vi "Dot_Plot_Sub.vi"(8 "Scaler plotted":string, 11 "Data":dbl[][](array[numeric])=[[-106.4208, 283.2907, 10.0, -0.027074, 202.4772, -73.9844, 9.9544], [-106.4108, 183.2989, 10.0, -0.06373, 202.4772, -73.9844, 9.9544], [-106.4104, 233.2978, 10.0, -0.10129, 202.4772, -73.9844, 9.9544], [-106.408, 333.302, 10.0, -0.09306, 202.4772, -73.9844, 9.9544], [138.8906, 606.731, 10.0, -0.003285, 202.4772, -73.9844, 9.9544], [238.889, 47.6577, 10.0, 0.004673, 202.4772, -73.9844, 9.9544], [238.8902, 606.729, 10.0, -0.003458, 202.4772, -73.9844, 9.9544], [288.8878, 47.6581, 10.0, 0.007221, 202.4772, -73.9844, 9.9544], [338.888, 606.73, 10.0, 0.004362, 202.4772, -73.9844, 9.9544], [338.891, 47.6626, 10.0, 0.006298, 202.4772, -73.9844, 9.9544], [388.892, -63.3583, 10.0, 4.5324, 202.4772, -73.9844, 9.9544], [388.892, 47.6606, 10.0, -0.008191, 202.4772, -73.9844, 9.9544], [438.889, 606.729, 10.0, -0.0028755, 202.4772, -73.9844, 9.9544], [438.89, -63.3577, 10.0, 4.2681, 202.4772, -73.9844, 9.9544], [438.891, 47.6608, 10.0, 0.026059, 202.4772, -73.9844, 9.9544], [488.89, 47.6614, 10.0, 0.14972, 202.4772, -73.9844, 9.9544], [488.892, -63.3599, 10.0, 6.2235, 202.4772, -73.9844, 9.9544], [538.89, -63.3596, 10.0, 7.0971, 202.4772, -73.9844, 9.9544], [538.891, 47.6597, 10.0, 0.7831, 202.4772, -73.9844, 9.9544], [538.893, 606.731, 10.0, 0.004097, 202.4772, -73.9844, 9.9544], [588.889, -63.3589, 10.0, 9.8267, 202.4772, -73.9844, 9.9544], [588.89, 47.659, 10.0, 1.4958, 202.4772, -73.9844, 9.9544], [638.889, 47.6597, 10.0, 2.7164, 202.4772, -73.9844, 9.9544], [638.89, 606.731, 10.0, 0.0016489, 202.4772, -73.9844, 9.9544], [638.891, -63.361, 10.0, 9.6904, 202.4772, -73.9844, 9.9544], [688.89, -63.3603, 10.0, 10.7752, 202.4772, -73.9844, 9.9544], [688.89, 47.6576, 10.0, 4.0933, 202.4772, -73.9844, 9.9544], [738.888, -63.3603, 10.0, 9.798, 202.4772, -73.9844, 9.9544], [738.889, 47.6583, 10.0, 5.4641, 202.4772, -73.9844, 9.9544], [738.89, 606.73, 10.0, 0.03667, 202.4772, -73.9844, 9.9544], [788.888, 47.659, 10.0, 6.5562, 202.4772, -73.9844, 9.9544], [788.889, -63.3624, 10.0, 9.7284, 202.4772, -73.9844, 9.9544], [838.888, -63.3617, 10.0, 9.2828, 202.4772, -73.9844, 9.9544], [838.888, 606.731, 10.0, 0.10792, 202.4772, -73.9844, 9.9544], [838.889, 47.6562, 10.0, 6.9452, 202.4772, -73.9844, 9.9544], [888.892, 47.6611, 10.0, 6.813, 202.4772, -73.9844, 9.9544], [888.892, -63.3575, 10.0, 8.8351, 202.4772, -73.9844, 9.9544], [938.888, 606.729, 10.0, 0.5974, 202.4772, -73.9844, 9.9544], [938.891, 47.6618, 10.0, 5.8719, 202.4772, -73.9844, 9.9544], [938.892, -63.3596, 10.0, 8.3492, 202.4772, -73.9844, 9.9544], [988.889, 47.6618, 10.0, 4.8748, 202.4772, -73.9844, 9.9544], [988.891, -63.3589, 10.0, 7.5502, 202.4772, -73.9844, 9.9544], [1038.888, 297.6587, 10.0, 3.1165, 202.4772, -73.9844, 9.9544], [1038.888, 97.6613, 10.0, 4.0692, 202.4772, -73.9844, 9.9544], [1038.888, 222.6594, 10.0, 2.9843, 202.4772, -73.9844, 9.9544], [1038.889, 147.6602, 10.0, 3.7073, 202.4772, -73.9844, 9.9544], [1038.889, 272.6583, 10.0, 3.0147, 202.4772, -73.9844, 9.9544], [1038.89, 72.6609, 10.0, 4.1188, 202.4772, -73.9844, 9.9544], [1038.89, 122.659, 10.0, 3.9763, 202.4772, -73.9844, 9.9544], [1038.89, 197.659, 10.0, 3.099, 202.4772, -73.9844, 9.9544], [1038.89, 247.6571, 10.0, 2.9194, 202.4772, -73.9844, 9.9544], [1038.89, 322.657, 10.0, 2.9534, 202.4772, -73.9844, 9.9544], [1038.89, 572.66, 10.0, 1.2565, 202.4772, -73.9844, 9.9544], [1038.89, 172.6578, 10.0, 3.3414, 202.4772, -73.9844, 9.9544], [1038.89, 447.662, 10.0, 2.4811, 202.4772, -73.9844, 9.9544], [1038.89, 522.662, 10.0, 1.3205, 202.4772, -73.9844, 9.9544], [1038.89, 47.6597, 10.0, 4.5287, 202.4772, -73.9844, 9.9544], [1038.89, -63.3589, 10.0, 6.8815, 202.4772, -73.9844, 9.9544], [1038.891, 372.662, 10.0, 2.8557, 202.4772, -73.9844, 9.9544], [1038.891, 497.66, 10.0, 1.5334, 202.4772, -73.9844, 9.9544], [1038.891, 547.66, 10.0, 1.2132, 202.4772, -73.9844, 9.9544], [1038.892, 422.661, 10.0, 2.7183, 202.4772, -73.9844, 9.9544], [1038.892, 472.661, 10.0, 1.9636, 202.4772, -73.9844, 9.9544], [1038.893, -7.8602, 10.0, 4.95, 202.4772, -73.9844, 9.9544], [1038.893, 347.662, 10.0, 2.9008, 202.4772, -73.9844, 9.9544], [1038.893, 606.731, 10.0, 1.1868, 202.4772, -73.9844, 9.9544], [1038.893, 397.661, 10.0, 2.8316, 202.4772, -73.9844, 9.9544], [1138.89, 606.732, 10.0, 1.4995, 202.4772, -73.9844, 9.9544], [1238.891, 606.73, 10.0, 1.7166, 202.4772, -73.9844, 9.9544], [1338.89, 606.729, 10.0, 1.8307, 202.4772, -73.9844, 9.9544], [1438.888, 606.729, 10.0, 1.8125, 202.4772, -73.9844, 9.9544]]) -> ()   [LabVIEW 2021]
uses:
  <vilib>/Utility/miscctls.llb/LV3DPointTypeDef.ctl
  <vilib>/Utility/miscctls.llb/LVRGBAColorTypeDef.ctl
  <vilib>/picture/3D Picture Control/Object/Create Object (drawable).vi
  <vilib>/picture/3D Picture Control/Object/Add Object (reference).vi
  Gen Trav/Route mapping/Route_mapping_global.vi
  <vilib>/picture/3D Picture Control/Helpers/Set Light (no reference).vi
  Globals/Constants_global.vi
  <vilib>/picture/3D Picture Control/NI_3D Picture Control.lvlib
panel:
  in  "Font, Size & Style":T1={"Desired Font (Application)"=enum."User-specified Font", "[User-specified Font]"={"Font Name"="Arial", "Size"=18, "Strikeout?"=FALSE, "Italic?"=FALSE, "Underline?"=FALSE, "Outline?"=FALSE, "Shadow?"=FALSE, "Bold?"=FALSE, "Rotation Angle"=0.0}, "Horizontal Alignment"=1, "Vertical Alignment"=0} {"Vertical Alignment" items=["Bottom", "Top", "Baseline"]; "Horizontal Alignment" items=["Left", "Center", "Right"]; "[User-specified Font]"."Rotation Angle" format="%.2f"}
  in  "Text position":u16(ring) items=["Top", "Bottom"]
  in  "Path to save picture":path=path "C:/Users/Paul Nathan/Desktop/test.jpg"
  in  "Save Picture":bool
  in  "Lift Measurement Position":dbl
  in  "Camera Position":T2={"X"=-0.0, "Y"=0.001, "Z"=3000.0}
  in  "Auto Camera Position":bool=TRUE
  in  "Bar Plot":bool
  in  "Max column Height":i32=1000
  in  "Manual Range":bool
  in  "Dem Min":dbl
  in  "Dem Max":dbl
  out "min value":dbl=-0.10129
  out "max value":dbl=10.7752
  in  "stop":bool
  in  "Space File Opacity":dbl(slide)=0.5051546391752577 scale=0.0..1.0
  in  "STL Model Opacity":dbl(slide)=1.0 scale=0.0..1.0
  in  "Fixed Colour":u32(colorbox)=16860
  in  "Cube Size":sgl=20.0
  in  "Model rotation":sgl(knob) scale=-360.0..360.0
  in  "Camera Height":dbl(slide)=3000.0 scale=1000.0..5000.0
  in  "Y shift":dbl(slide) scale=-3000.0..3000.0
  in  "X shift":sgl(slide) scale=-3000.0..3000.0
  in  "Model rotation axis":cluster{"X":sgl, "Y":sgl, "Z":sgl}={"X"=0.0, "Y"=0.0, "Z"=1.0}
  in  "Lock to plan view":bool=TRUE
  in  "Up Direction":T2={"X"=0.0, "Y"=0.0, "Z"=1.0}
  in  "Target":T2={"X"=-0.0, "Y"=-0.0, "Z"=0.0}
  in  "Browse CAD Model":path=path "C:/EnFlo Software/Anemometry/Anemometry Sub Vis/Templates/Diplos2.stl"
  in  "STL Model Colour":u32(colorbox)=16448250
  in  "Measurement\n Color Ramp":u32[](array[colorbox])=[16711680, 16776960, 6618880, 0]
  in  "Radius":sgl=20.0
  in  "Space File Color":u32(colorbox)=9868950
  out "3D Picture Control":refnum<vi>(3d-picture)
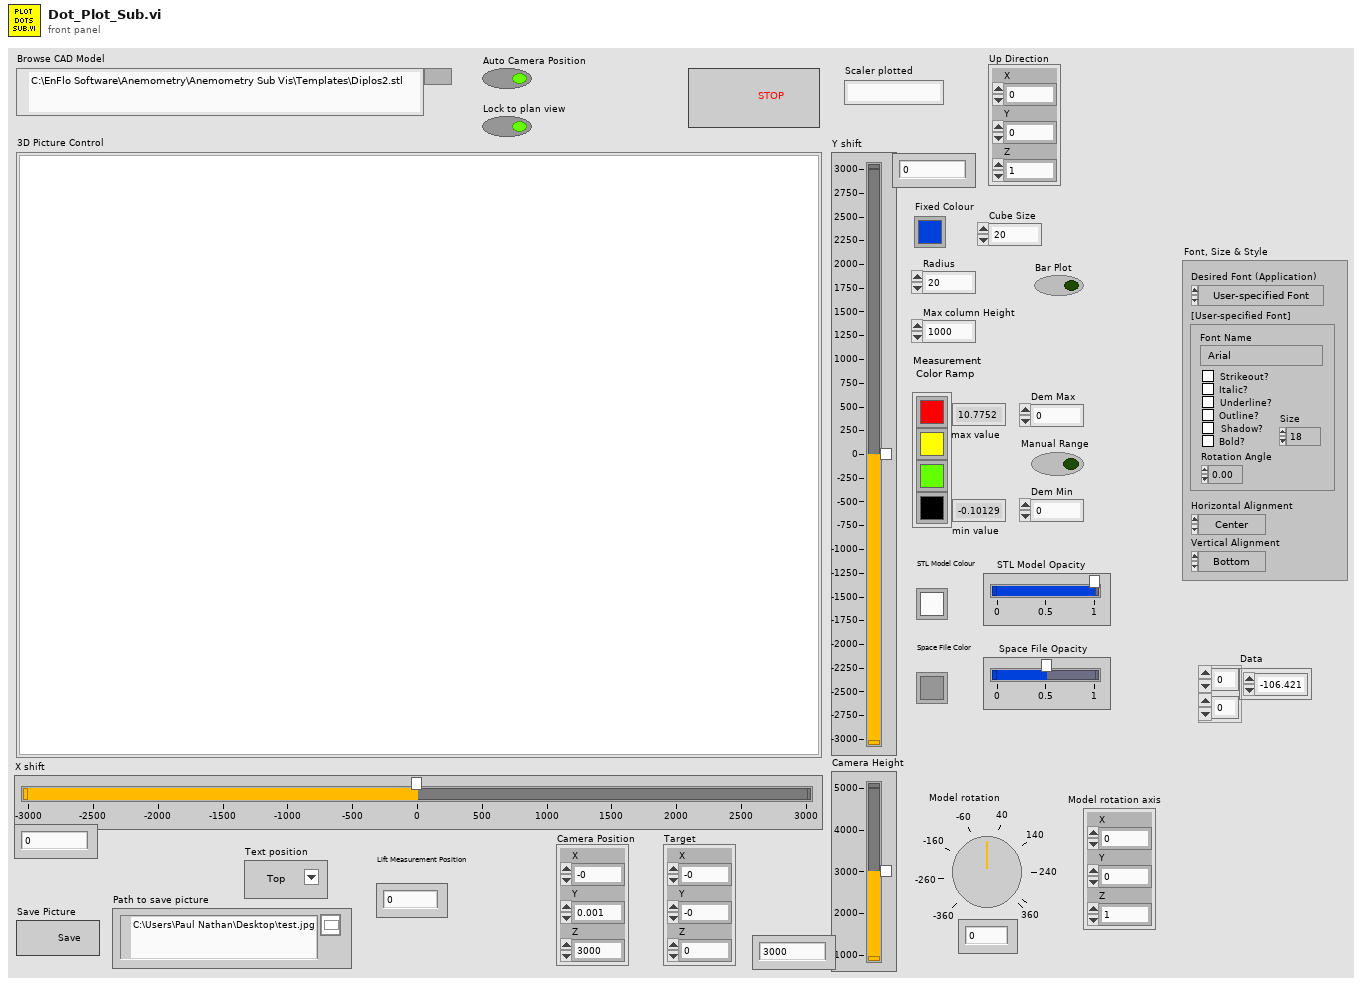
[diagram p1: front panel]
types:
  T1 = cluster{"Desired Font (Application)":enum16{"User-specified Font", "Application Font", "System Font", "Dialog Font"}, "[User-specified Font]":cluster{"Font Name":string, "Size":i16, "Strikeout?":bool, "Italic?":bool, "Underline?":bool, "Outline?":bool, "Shadow?":bool, "Bold?":bool, "Rotation Angle":dbl}, "Horizontal Alignment":i16, "Vertical Alignment":i16}
  T2 = typedef "LV3DPointTypeDef.ctl" = cluster{"X":sgl, "Y":sgl, "Z":sgl}
  T3 = enum16{"Inherit Value", "Points", "Wireframe", "Polygons"}
  T4 = enum16{"Inherit Value", "No Culling", "Cull Back Face", "Cull Front Face", "Cull Both Faces"}
  T5 = enum16{"Inherit Value", "Counterclockwise", "Clockwise"}
  T6 = typedef "LVRGBAColorTypeDef.ctl" = cluster{"Red":sgl, "Green":sgl, "Blue":sgl, "Alpha":sgl}
  T7 = typedef "Triangle.ctl" = cluster{"V0":sgl[], "V1":sgl[], "V2":sgl[], "E0":sgl[], "E1":sgl[], "E2":sgl[], "n^":sgl[], "nE0^":sgl[], "nE1^":sgl[], "nE2^":sgl[]}
  T8 = typedef "Exclude_cluster.ctl" = cluster{"Sizes":T9, "Name":string, "Exclude Type":T10}
  T9 = typedef "Box_size.ctl" = cluster{"Max":sgl, "Min":sgl}[]
  T10 = typedef "Exclusion_type.ctl" = enum16{"Exclude completely", "Allow only vertical moves"}
  T11 = typedef "imagedata.ctl" = cluster{"image type":i32, "image depth":i32, "image":u8[], "mask":u8[], "colors":u32[], "Rectangle":cluster{"left":i16, "top":i16, "right":i16, "bottom":i16}}
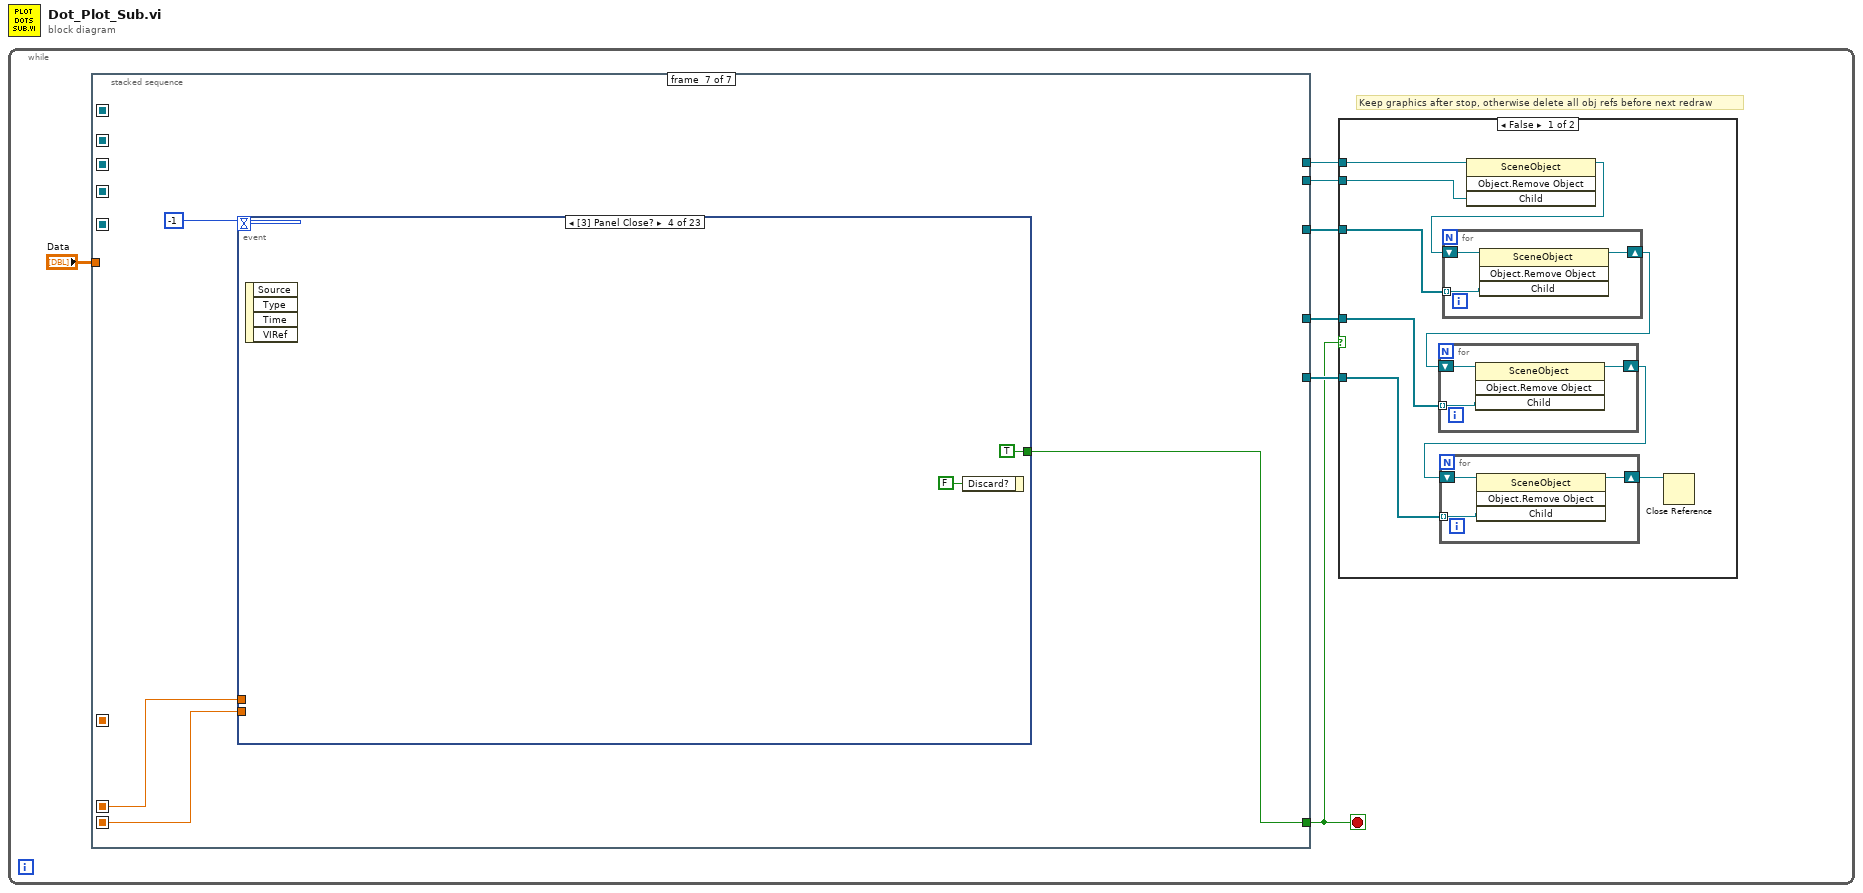
[diagram p0: block diagram]
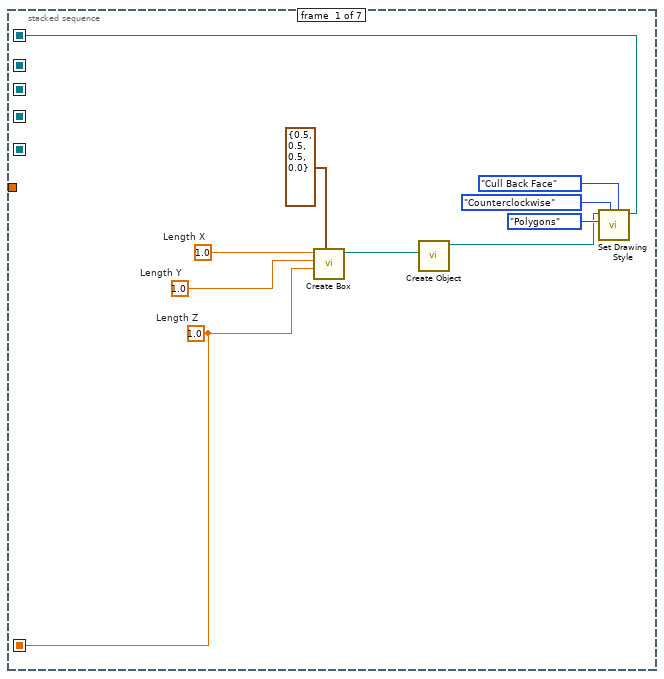
[diagram p3: hidden frame]
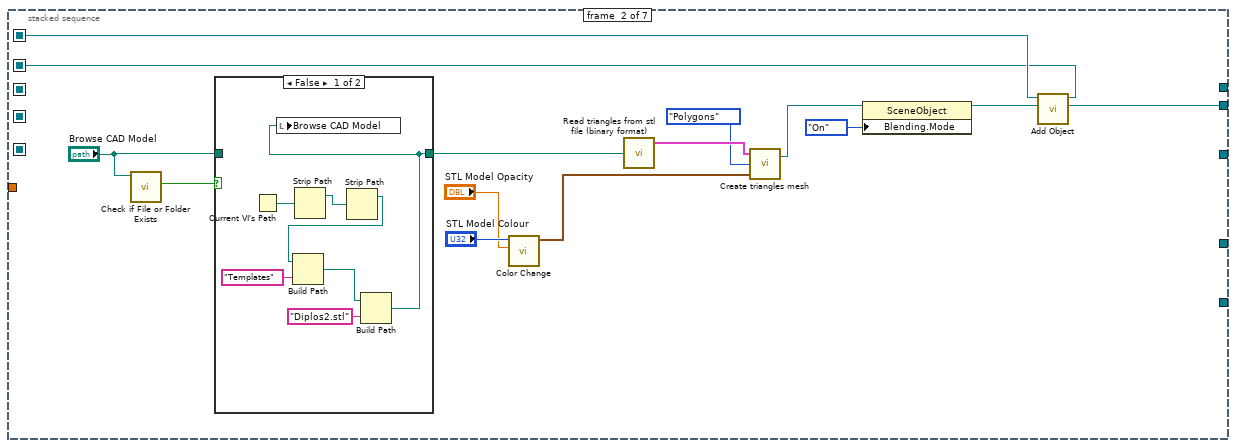
[diagram p4: hidden frame]
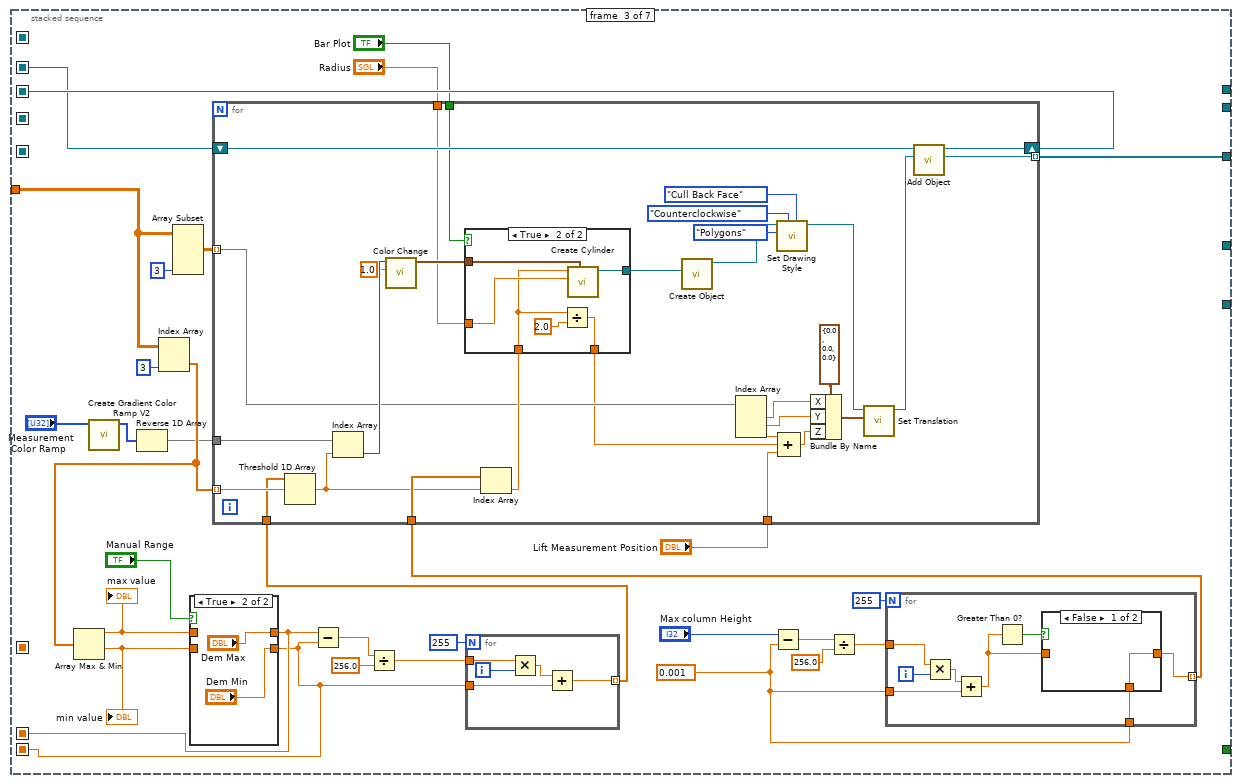
[diagram p6: hidden frame]
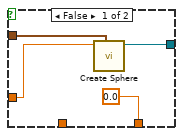
[diagram p9: hidden frame]
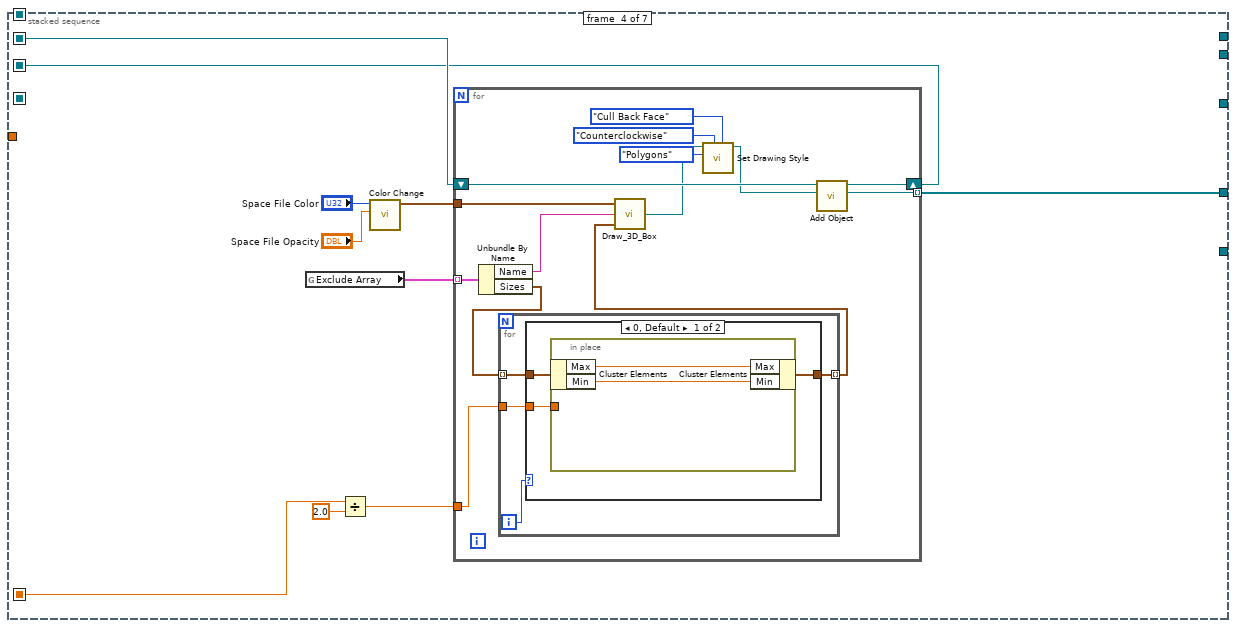
[diagram p10: hidden frame]
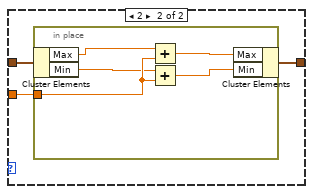
[diagram p11: hidden frame]
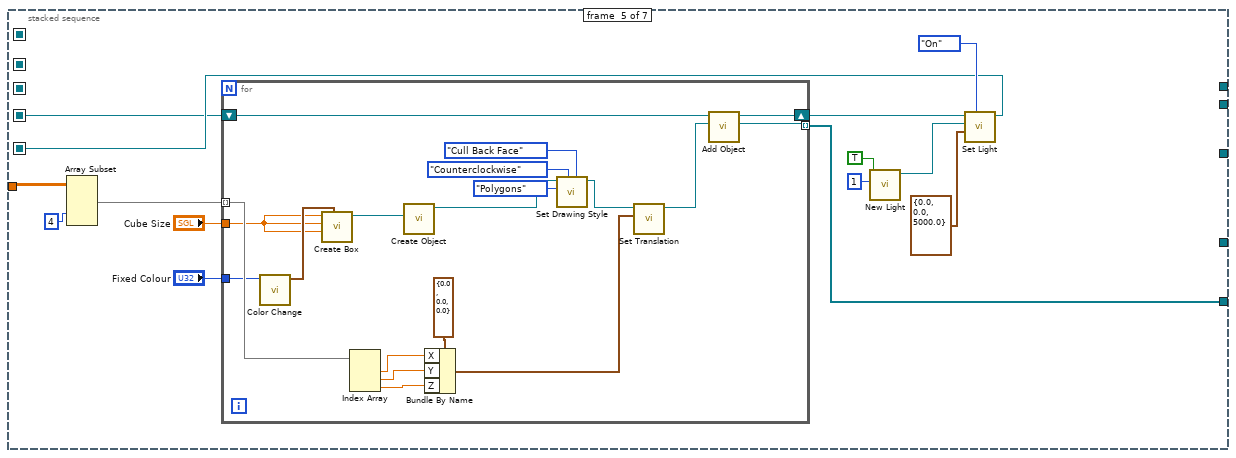
[diagram p12: hidden frame]
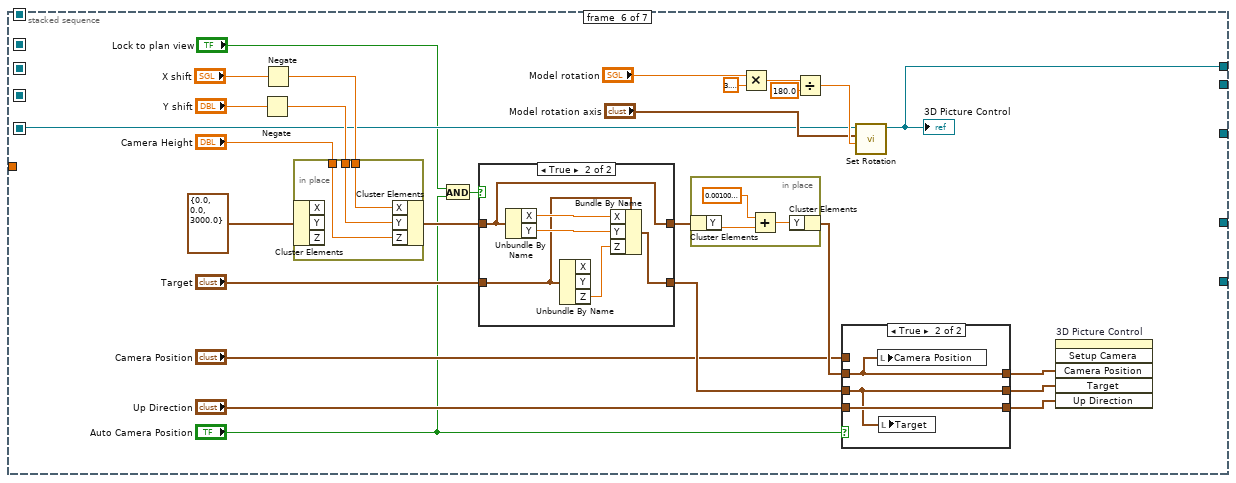
[diagram p13: hidden frame]
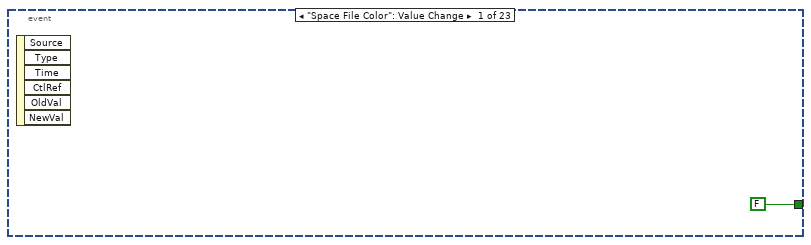
[diagram p16: hidden frame]
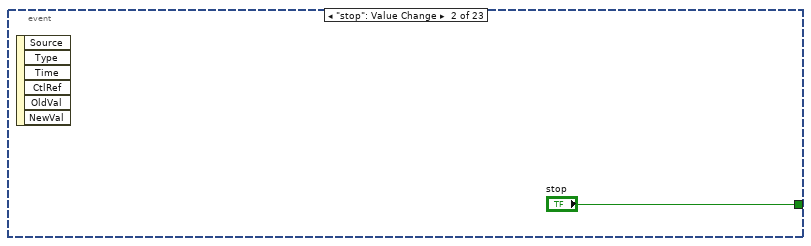
[diagram p17: hidden frame]
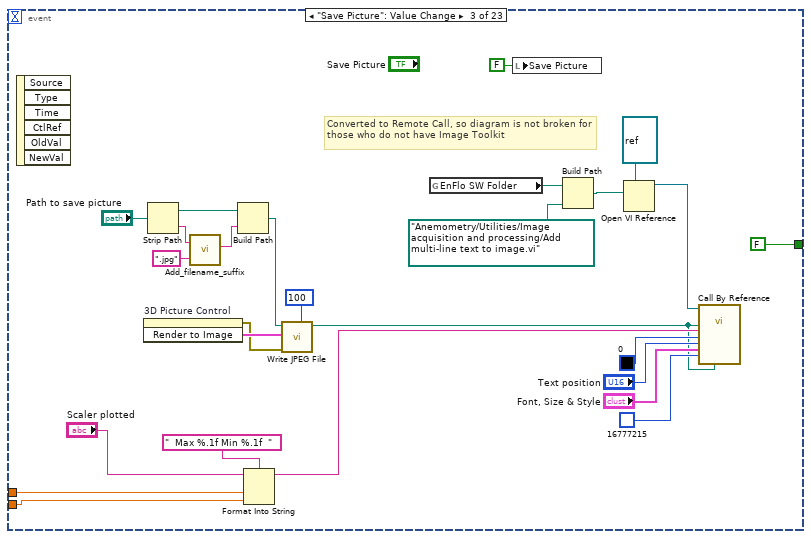
[diagram p18: hidden frame]
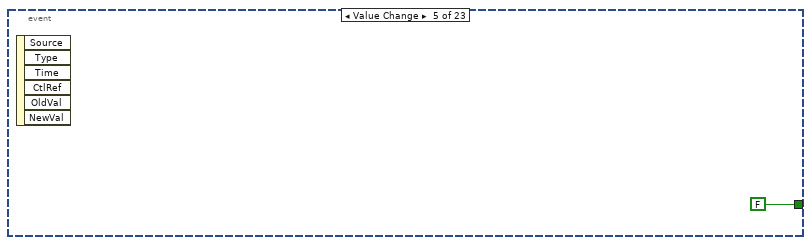
[diagram p19: hidden frame]
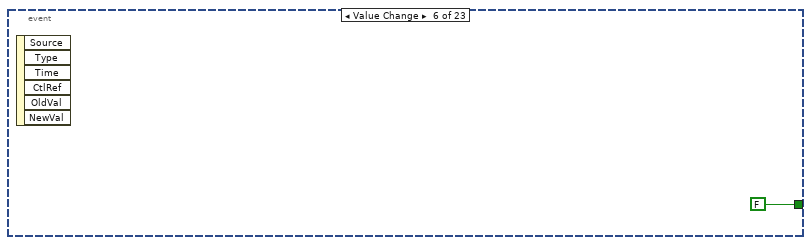
[diagram p20: hidden frame]
diagram:
  n1 = while {
    stop <- w1 stop-if-true
    # "Keep graphics after stop, otherwise delete all obj refs before next redraw"
    n2 = stacked-sequence {
      seq-local: [w26 _ _ _ _ _ _] -> [_ w49 _ _ _ _ _]
      seq-local: [w35 _ _ _ _ _ _] -> [_ _ _ w151 _ _ _]
      seq-local: [_ w48 _ _ _ _ _] -> [_ _ w75 _ _ _ _]
      seq-local: [_ _ w76 _ _ _ _] -> [_ _ _ w153 _ _ _]
      seq-local: [_ _ _ _ w193 _ _] -> [_ _ _ _ _ w231 _]
      seq-local: [_ _ _ w152 _ _ _] -> [_ _ _ _ w192 _ _]
      seq-local: [_ _ w59 _ _ _ _] -> [_ _ _ _ _ _ w270]
      seq-local: [_ _ w58 _ _ _ _] -> [_ _ _ _ _ _ w269]
      tunnel: "Data" -> [_ _ w79 _ w196 _ _]
      tunnel: [_ _ _ _ _ _ w272] -> w1
      tunnel: [_ w36 _ _ _ _ _] -> w5
      tunnel: [_ _ w63 _ _ _ _] -> w6
      tunnel: [_ _ _ w148 _ _ _] -> w3
      tunnel: [_ _ _ _ w191 _ _] -> w2
      tunnel: [_ _ _ _ _ w229 _] -> w4
      frame #0 {
        w35 = sgl 1.0  # Length Z
        w32 = sgl 1.0  # Length Y
        w33 = sgl 1.0  # Length X
        n3 = call <vilib>:"Create Box.vi"("Color"=T6 {"Red"=0.5, "Green"=0.5, "Blue"=0.5, "Alpha"=0.0} ("Color 2"), "Length Z"=w35, "Length Y"=w32, "Length X"=w33) -> ("New Box Refnum"=w31:refnum<vi>)  [unwired: 6 in, 1 out]
        n4 = call-poly <vilib>:"Create Object.vi"("Geometry"=w31) -> ("Scene:New Object"=w27:refnum<vi>)  [unwired: 9 in, 1 out]
        n5 = call <vilib>:"Set Drawing Style.vi"("Face Culling Mode"=T4."Cull Back Face", "Frontface Mode"=T5."Counterclockwise", "Mode"=T3."Polygons", "Scene Object In"=w27) -> ("Scene Object Out"=w26:refnum<vi>)  [unwired: 6 in, 1 out]
      }
      frame #1 {
        n6 = call <vilib>:"Check if File or Folder Exists.vi"("path"="Browse CAD Model") -> ("file or folder exists?"=w46:bool)  [unwired: 8 in, 2 out]
        n7 = case shown="False" w46 {
          tunnel: [w50 w57] -> w42
          tunnel: "Browse CAD Model" -> [_ w57]
          frame False {
            n8 = Current VI's Path() -> (path=w56:path)
            n9 = Strip Path(path=w56) -> (stripped path=w55:path)  [unwired: 1 out]
            n10 = Strip Path(path=w55) -> (stripped path=w54:path)  [unwired: 1 out]
            n11 = Build Path(base path=w54, name or relative path="Templates") -> (appended path=w52:path)
            n12 = Build Path(base path=w52, name or relative path="Diplos2.stl") -> (appended path=w50:path)
            n13 = local write "Browse CAD Model"(w50) -> ()
          }
          frame True {
          }
        }
        n14 = call <vilib>:"Color Change.vi"("Alpha"="STL Model Opacity", "Color"="STL Model Colour") -> ("RGBA"=w39:cluster{"R":sgl, "G":sgl, "B":sgl, "A":sgl})  [unwired: 9 in]
        n15 = call "Read triangles from stl file (binary format).vi"("STL file path"=w42) -> ("Triangles array"=w41:T7[])  [unwired: 2 out]
        n16 = call "Create triangles mesh.vi"("Colour"=w39, "Render mode"=T3."Polygons", "Triangles array"=w41) -> ("Triangle mesh out"=w37:refnum<vi>)  [unwired: 1 out]
        n17 = property class="SceneObject"(reference=w37, "Blending.Mode"=enum16{"Inherit Value", "Off", "On"}."On" ("Blending:Mode")) -> (reference out=w43:refnum<vi>)  [unwired: 1 in, 1 out]
        n18 = call-poly <vilib>:"Add Object.vi"("New Object In"=w43, "Scene Object In"=w49) -> ("New Object Out"=w36:refnum<vi>, "Scene Object Out"=w48:refnum<vi>)  [unwired: 7 in, 1 out]
      }
      frame #2 {
        w66 = 0.001
        n19 = call "Create Gradient Color Ramp V2.vi"("Color Array"="Measurement\n Color Ramp") -> ("Color Table"=w87:u32[])  [unwired: 10 in]
        n20 = Reverse 1D Array(array=w87) -> (reversed array=w84:u32[])
        n21 = Index Array(array=w79, index (col)=3 ("disabled index (col)")) -> (element=w85:dbl[])  [unwired: 1 in]
        n22 = Array Max & Min(array=w85) -> (max value=w73:dbl, min value=w72:dbl)  [unwired: 2 out]
        "max value" <- w73
        "min value" <- w72
        n23 = Array Subset(array=w79, length (col)=3 ("length")) -> (w77:dbl[][])  [unwired: 3 in]
        n24 = case shown="True" "Manual Range" {
          tunnel: [w100 "Dem Max"] -> w59
          tunnel: w73 -> [w100 _]
          tunnel: [w99 "Dem Min"] -> w58
          tunnel: w72 -> [w99 _]
          frame False {
          }
          frame True {
          }
        }
        n25 = Subtract(x=w59, y=w58) -> (x-y=w83:dbl)
        n26 = Divide(x=w83, y=256.0) -> (x/y=w81:dbl)
        n27 = for {
          N: 255 -> [_]
          tunnel: w81 -> [w106]
          tunnel: w58 -> [w104]
          tunnel: [w103] -> w65 mode=indexing
          i -> [w107]
          n28 = Multiply(x=w106, y=w107) -> (x*y=w105:dbl)
          n29 = Add(x=w105, y=w104) -> (x+y=w103:dbl)
        }
        n30 = Subtract(x="Max column Height", y=w66) -> (x-y=w68:dbl)
        n31 = Divide(x=w68, y=256.0) -> (x/y=w70:dbl)
        n32 = for {
          N: 255 -> [_]
          tunnel: w70 -> [w95]
          tunnel: w66 -> [w93]
          tunnel: [w92] -> w67 mode=indexing
          tunnel: w66 -> [w89]
          i -> [w96]
          n33 = Multiply(x=w95, y=w96) -> (x*y=w94:dbl)
          n34 = Add(x=w94, y=w93) -> (x+y=w91:dbl)
          n35 = Greater Than 0?(x=w91) -> (x > 0?=w90:bool)
          n36 = case shown="False" w90 {
            tunnel: [w97 w98] -> w92
            tunnel: w91 -> [_ w98]
            tunnel: w89 -> [w97 _]
            frame False {
            }
            frame True {
            }
          }
        }
        n37 = for {
          shift-right: [w132] -> w76
          shift-left: w75 -> [w133]
          tunnel: w67 -> [w127]
          tunnel: w85 -> [w125] mode=indexing
          tunnel: w84 -> [w126]
          tunnel: w77 -> [w123] mode=indexing
          tunnel: w65 -> [w124]
          tunnel: [w117] -> w63 mode=indexing
          tunnel: "Bar Plot" -> [w110]
          tunnel: "Radius" -> [w109]
          tunnel: "Lift Measurement Position" -> [w108]
          n38 = Threshold 1D Array(2:w125, 3:w124) -> (0:w122:dbl)  [unwired: 1 in]
          n39 = Index Array(array=w126, index=w122) -> (element=w129:u32)
          n40 = call <vilib>:"Color Change.vi"("Alpha"=1.0, "Color"=w129) -> ("RGBA"=w130:cluster{"R":sgl, "G":sgl, "B":sgl, "A":sgl})  [unwired: 9 in]
          n41 = Index Array(array=w127, index=w122) -> (element=w128:dbl)
          n42 = case shown="True" w110 {
            tunnel: w130 -> [w140 w147]
            tunnel: [w139 w146] -> w118
            tunnel: w109 -> [w141 w145]
            tunnel: w128 -> [_ w142]
            tunnel: [0.0 w143] -> w119
            frame False {
              n43 = call <vilib>:"Create Sphere.vi"("Color"=w140, "Radius"=w141) -> ("New Sphere Refnum"=w139:refnum<vi>)  [unwired: 8 in, 1 out]
            }
            frame True {
              n44 = Divide(x=w142, y=2.0) -> (x/y=w143:dbl)
              n45 = call <vilib>:"Create Cylinder.vi"("Color"=w147, "Radius"=w145, "Height"=w142) -> ("New Cylinder Refnum"=w146:refnum<vi>)  [unwired: 7 in, 1 out]
            }
          }
          n46 = call-poly <vilib>:"Create Object.vi"("Geometry"=w118) -> ("Scene:New Object"=w115:refnum<vi>)  [unwired: 9 in, 1 out]
          n47 = Index Array(array=w123) -> (element #1=w136:dbl, element #2=w137:dbl, element #3=w121:dbl)  [unwired: 3 in]
          n48 = call <vilib>:"Set Drawing Style.vi"("Face Culling Mode"=T4."Cull Back Face", "Frontface Mode"=T5."Counterclockwise", "Mode"=T3."Polygons", "Scene Object In"=w115) -> ("Scene Object Out"=w114:refnum<vi>)  [unwired: 6 in, 1 out]
          n49 = Compound Arithmetic op=ADD(w121, w119, w108) -> (w120:dbl)
          n50 = Bundle By Name(cluster=cluster{"X":sgl, "Y":sgl, "Z":sgl} {"X"=0.0, "Y"=0.0, "Z"=0.0} ("Translation"), "X"=w136, "Y"=w137, "Z"=w120) -> (w134:cluster{"X":sgl, "Y":sgl, "Z":sgl})
          n51 = call <vilib>:"Set Translation.vi"("Translation"=w134, "Scene Object"=w114) -> ("Translated Object"=w131:refnum<vi>)  [unwired: 8 in, 1 out]
          n52 = call-poly <vilib>:"Add Object.vi"("New Object In"=w131, "Scene Object In"=w133) -> ("New Object Out"=w117:refnum<vi>, "Scene Object Out"=w132:refnum<vi>)  [unwired: 7 in, 1 out]
        }
      }
      frame #3 {
        n53 = global read "Route_mapping_global.vi" "Exclude Array"() -> (w157:T8[])
        n54 = Divide(x=w151, y=sgl 2.0) -> (x/y=w154:sgl)
        n55 = call <vilib>:"Color Change.vi"("Alpha"="Space File Opacity", "Color"="Space File Color") -> ("RGBA"=w149:cluster{"R":sgl, "G":sgl, "B":sgl, "A":sgl})  [unwired: 9 in]
        n56 = for {
          tunnel: w157 -> [w171] mode=indexing
          tunnel: w149 -> [w170]
          tunnel: w154 -> [w168]
          shift-right: [w164] -> w152
          shift-left: w153 -> [w165]
          tunnel: [w163] -> w148 mode=indexing
          n57 = Unbundle By Name(w171) -> ("Name"=w169:string, "Sizes"=w167:T9)
          n58 = for {
            tunnel: w168 -> [w175]
            tunnel: w167 -> [w174] mode=indexing
            tunnel: [w173] -> w166 mode=indexing
            i -> [w172]
            n59 = case shown="0, Default" w172 {
              tunnel: w175 -> [w178 w183]
              tunnel: w174 -> [w177 w182]
              tunnel: [w176 w181] -> w173
              frame 0, Default {
                n60 = in-place {
                  in-place-border: w178 -> [_]
                  n61 = in-place-cluster #1(w177) -> ("Max"=w180:sgl, "Min"=w179:sgl)
                  n62 = in-place-cluster #1("Max"=w180, "Min"=w179) -> (w176:cluster{"Max":sgl, "Min":sgl})
                }
              }
              frame 2 {
                n63 = in-place {
                  in-place-border: w183 -> [w188]
                  n64 = in-place-cluster #2(w182) -> ("Max"=w185:sgl, "Min"=w184:sgl)
                  n65 = Add(x=w185, y=w188) -> (x+y=w187:sgl)
                  n66 = Add(x=w184, y=w188) -> (x+y=w186:sgl)
                  n67 = in-place-cluster #2("Max"=w187, "Min"=w186) -> (w181:cluster{"Max":sgl, "Min":sgl})
                }
              }
            }
          }
          n68 = call "Draw_3D_Box.vi"("Box Coordinates"=w166, "Name"=w169, "Color"=w170) -> ("Translated Object"=w159:refnum<vi>)
          n69 = call <vilib>:"Set Drawing Style.vi"("Face Culling Mode"=T4."Cull Back Face", "Frontface Mode"=T5."Counterclockwise", "Mode"=T3."Polygons", "Scene Object In"=w159) -> ("Scene Object Out"=w158:refnum<vi>)  [unwired: 6 in, 1 out]
          n70 = call-poly <vilib>:"Add Object.vi"("New Object In"=w158, "Scene Object In"=w165) -> ("New Object Out"=w163:refnum<vi>, "Scene Object Out"=w164:refnum<vi>)  [unwired: 7 in, 1 out]
        }
      }
      frame #4 {
        n71 = Array Subset(array=w196, index (col)=4 ("length")) -> (w195:dbl[][])  [unwired: 3 in]
        n72 = for {
          tunnel: w195 -> [w212] mode=indexing
          shift-right: [w215] -> w197
          shift-left: w192 -> [w216]
          tunnel: [w210] -> w191 mode=indexing
          tunnel: "Fixed Colour" -> [w204]
          tunnel: "Cube Size" -> [w203]
          n73 = call <vilib>:"Color Change.vi"("Color"=w204) -> ("RGBA"=w213:cluster{"R":sgl, "G":sgl, "B":sgl, "A":sgl})  [unwired: 10 in]
          n74 = call <vilib>:"Create Box.vi"("Color"=w213, "Length Z"=w203, "Length Y"=w203, "Length X"=w203) -> ("New Box Refnum"=w211:refnum<vi>)  [unwired: 6 in, 1 out]
          n75 = Index Array(array=w212) -> (element #1=w219:dbl, element #2=w220:dbl, element #3=w221:dbl)  [unwired: 3 in]
          n76 = call-poly <vilib>:"Create Object.vi"("Geometry"=w211) -> ("Scene:New Object"=w206:refnum<vi>)  [unwired: 9 in, 1 out]
          n77 = Bundle By Name(cluster=cluster{"X":sgl, "Y":sgl, "Z":sgl} {"X"=0.0, "Y"=0.0, "Z"=0.0} ("Translation"), "X"=w219, "Y"=w220, "Z"=w221) -> (w217:cluster{"X":sgl, "Y":sgl, "Z":sgl})
          n78 = call <vilib>:"Set Drawing Style.vi"("Face Culling Mode"=T4."Cull Back Face", "Frontface Mode"=T5."Counterclockwise", "Mode"=T3."Polygons", "Scene Object In"=w206) -> ("Scene Object Out"=w205:refnum<vi>)  [unwired: 6 in, 1 out]
          n79 = call <vilib>:"Set Translation.vi"("Translation"=w217, "Scene Object"=w205) -> ("Translated Object"=w214:refnum<vi>)  [unwired: 8 in, 1 out]
          n80 = call-poly <vilib>:"Add Object.vi"("New Object In"=w214, "Scene Object In"=w216) -> ("New Object Out"=w210:refnum<vi>, "Scene Object Out"=w215:refnum<vi>)  [unwired: 7 in, 1 out]
        }
        n81 = call <vilib>:"New Light.vi"("Light Number"=1, "At Infinity"=TRUE) -> ("New Light Refnum"=w199:refnum<vi>)  [unwired: 8 in, 1 out]
        n82 = call-poly <vilib>:"Set Light.vi"("Light State"=enum16{"Inherit Value", "Off", "On"}."On", "Position"=T2 {"X"=0.0, "Y"=0.0, "Z"=5000.0}, "Light Refnum In"=w199, "Scene Object In"=w197) -> ("Scene Object Out"=w193:refnum<vi>)  [unwired: 6 in, 1 out]
      }
      frame #5 {
        n83 = Negate(x="Y shift") -> (-x=w234:dbl)
        n84 = Negate(x="X shift") -> (-x=w235:sgl)
        n85 = in-place {
          in-place-border: w235 -> [w257]
          in-place-border: w234 -> [w256]
          in-place-border: "Camera Height" -> [w255]
          n86 = in-place-cluster #3(T2 {"X"=0.0, "Y"=0.0, "Z"=3000.0} ("Camera Position")) -> ()  [unwired: 3 out]
          n87 = in-place-cluster #3("X"=w257, "Y"=w256, "Z"=w255) -> (w238:T2)
        }
        n88 = And(x="Lock to plan view", y="Auto Camera Position") -> (x .and. y?=w223:bool)
        n89 = case shown="True" w223 {
          tunnel: w238 -> [w261 w263]
          tunnel: "Target" -> [w262 w266]
          tunnel: [w262 w264] -> w246
          tunnel: [w261 w263] -> w245
          frame False {
          }
          frame True {
            n90 = Unbundle By Name(w263) -> ("X"=w268:sgl, "Y"=w267:sgl)
            n91 = Unbundle By Name(w266) -> ("Z"=w265:sgl)  [unwired: 2 out]
            n92 = Bundle By Name(cluster=w266, "X"=w268, "Y"=w267, "Z"=w265) -> (w264:T2)
          }
        }
        n93 = in-place {
          n94 = in-place-cluster #4(w245) -> ("Y"=w260:sgl)
          n95 = Add(x=sgl 0.001, y=w260) -> (x+y=w259:sgl)
          n96 = in-place-cluster #4("Y"=w259) -> (w244:T2)
        }
        n97 = Multiply(x="Model rotation", y=sgl 3.1415927) -> (x*y=w243:sgl)
        n98 = Divide(x=w243, y=sgl 180.0) -> (x/y=w240:sgl)
        n99 = case shown="True" "Auto Camera Position" {
          tunnel: "Up Direction" -> [w251 w254]
          tunnel: w246 -> [w250 w252]
          tunnel: w244 -> [_ w253]
          tunnel: [w249 w253] -> w228
          tunnel: [w250 w252] -> w227
          tunnel: [w251 w254] -> w226
          tunnel: "Camera Position" -> [w249 _]
          frame False {
          }
          frame True {
            n100 = local write "Camera Position"(w253) -> ()
            n101 = local write "Target"(w252) -> ()
          }
        }
        n102 = call <vilib>:"Set Rotation.vi"("Angle"=w240, "Axis"="Model rotation axis", "Scene Object"=w231) -> ("Rotated Scene Object"=w229:refnum<vi>)  [unwired: 7 in, 1 out]
        "3D Picture Control" <- w229
        n103 = invoke on="3D Picture Control" class="SceneGraphDisp (strict)" method="Setup Camera"("Camera Position"=w228, "Target"=w227, "Up Direction"=w226) -> ()  [unwired: 3 in, 6 out]
      }
      frame #6 {
        n104 = event shown="[3] Panel Close?" {
          selector: _ -> [_ _ _ _ _ _ _ _ _ _ _ _ _ _ _ _ _ _ _ _ _ _ _]
          dyn-events: _ -> [_ _ _ _ _ _ _ _ _ _ _ _ _ _ _ _ _ _ _ _ _ _ _]
          timeout: -1 -> [_ _ _ _ _ _ _ _ _ _ _ _ _ _ _ _ _ _ _ _ _ _ _]
          tunnel: [FALSE ("stop") "stop" FALSE ("stop") TRUE ("stop") FALSE ("stop") FALSE ("stop") FALSE ("stop") FALSE ("stop") FALSE ("stop") FALSE ("stop") FALSE ("stop") FALSE ("stop") FALSE ("stop") FALSE ("stop") FALSE ("stop") FALSE ("stop") FALSE ("stop") FALSE ("stop") FALSE ("stop") FALSE ("stop") FALSE ("stop") FALSE ("stop") FALSE ("stop")] -> w272
          tunnel: w270 -> [_ _ w289 _ _ _ _ _ _ _ _ _ _ _ _ _ _ _ _ _ _ _ _]
          tunnel: w269 -> [_ _ w275 _ _ _ _ _ _ _ _ _ _ _ _ _ _ _ _ _ _ _ _]
          event "Space File Color": Value Change {
            n105 = event-data() -> ()  [unwired: 1 in, 6 out]
          }
          event "stop": Value Change {
            n106 = event-data() -> ()  [unwired: 1 in, 6 out]
          }
          event "Save Picture": Value Change {
            # "Converted to Remote Call, so diagram is not broken for those who do not have Image Toolkit"
            n107 = event-data() -> ()  [unwired: 1 in, 6 out]
            n108 = invoke on="3D Picture Control" class="SceneGraphDisp (strict)" method="Render to Image"() -> (error out=w299:errorcluster, "Get Image"=w300:T11)  [unwired: 3 in, 1 out]
            n109 = Strip Path(path="Path to save picture") -> (stripped path=w291:path, name=w293:string)
            n110 = call "Add_filename_suffix.vi"("Filename"=w293, "Suffix to add"=".jpg") -> ("Filename out"=w292:string)  [unwired: 3 out]
            n111 = Build Path(base path=w291, name or relative path=w292) -> (appended path=w290:path)
            n112 = Format Into String(format string="  Max %.1f Min %.1f  ", initial string="Scaler plotted", w289, w275) -> (resulting string=w278:string)  [unwired: 1 in, 1 out]
            n113 = call <vilib>:"Write JPEG File.vi"("quality (80)"=100, "error in (no error)"=w299, "image data"=w300, "path to JPEG file"=w290) -> ("path"=w277:path)  [unwired: 6 in, 1 out]
            n114 = global read "Constants_global.vi" "EnFlo SW Folder"() -> (w284:path)
            n115 = local write "Save Picture"(FALSE ("Save Picture")) -> ()
            n116 = Build Path(base path=w284, name or relative path=path "Anemometry/Utilities/Image acquisition and processing/Add multi-line text to image.vi") -> (appended path=w287:path)
            n117 = Open VI Reference(type specifier VI Refnum (for type only)=refnum<vi> refnum, vi path=w287) -> (vi reference=w286:refnum<vi>)  [unwired: 2 in, 3 out]
            n118 = call-by-ref "?"(reference=w286, "Text to add"=w278, "Image load path"=w277, "Text colour"=u32 0, "Text position"="Text position", "Font, Size & Style"="Font, Size & Style", "Background colour"=u32 16777215, "Image save path"=w277) -> ()  [unwired: 9 in, 3 out]
          }
          event Panel Close? {
            n119 = event-data() -> ()  [unwired: 1 in, 4 out]
            n120 = event-data("Discard?"=FALSE) -> ()  [unwired: 1 in, 1 out]
          }
          event Value Change {
            n121 = event-data() -> ()  [unwired: 1 in, 6 out]
          }
          event Value Change {
            n122 = event-data() -> ()  [unwired: 1 in, 6 out]
          }
          event Timeout {
            n123 = event-data() -> ()  [unwired: 1 in, 3 out]
          }
          event "Radius": Value Change {
            n124 = event-data() -> ()  [unwired: 1 in, 6 out]
          }
          event "Measurement\n Color Ramp": Value Change {
            n125 = event-data() -> ()  [unwired: 1 in, 6 out]
          }
          event "STL Model Colour": Value Change {
            n126 = event-data() -> ()  [unwired: 1 in, 6 out]
          }
          event "Lock to plan view": Value Change {
            n127 = event-data() -> ()  [unwired: 1 in, 6 out]
          }
          event "X shift": Value Change {
            n128 = event-data() -> ()  [unwired: 1 in, 6 out]
          }
          event "Y shift": Value Change {
            n129 = event-data() -> ()  [unwired: 1 in, 6 out]
          }
          event "Camera Height": Value Change {
            n130 = event-data() -> ()  [unwired: 1 in, 6 out]
          }
          event "Bar Plot": Value Change {
            n131 = event-data() -> ()  [unwired: 1 in, 6 out]
          }
          event "Auto Camera Position": Value Change {
            n132 = event-data() -> ()  [unwired: 1 in, 6 out]
          }
          event "Model rotation": Value Change {
            n133 = event-data() -> ()  [unwired: 1 in, 6 out]
          }
          event "STL Model Opacity": Value Change {
            n134 = event-data() -> ()  [unwired: 1 in, 6 out]
          }
          event "Space File Opacity": Value Change {
            n135 = event-data() -> ()  [unwired: 1 in, 6 out]
          }
          event "Dem Max": Value Change {
            n136 = event-data() -> ()  [unwired: 1 in, 6 out]
          }
          event "Dem Min": Value Change {
            n137 = event-data() -> ()  [unwired: 1 in, 6 out]
          }
          event "Manual Range": Value Change {
            n138 = event-data() -> ()  [unwired: 1 in, 6 out]
          }
          event "Cube Size": Value Change {
            n139 = event-data() -> ()  [unwired: 1 in, 6 out]
          }
        }
      }
    }
    n140 = case shown="False" w1 {
      tunnel: w6 -> [w16 _]
      tunnel: w5 -> [w15 _]
      tunnel: w4 -> [w14 _]
      tunnel: w3 -> [w12 _]
      tunnel: w2 -> [w10 _]
      frame False {
        n141 = invoke class="SceneObject" method="Object.Remove Object"(reference=w14, "Child"=w15) -> (reference out=w13:refnum<vi>)  [unwired: 2 in, 3 out]
        n142 = for {
          tunnel: w16 -> [w25] mode=indexing
          shift-right: [w23] -> w11
          shift-left: w13 -> [w24]
          n143 = invoke class="SceneObject" method="Object.Remove Object"(reference=w24, "Child"=w25) -> (reference out=w23:refnum<vi>)  [unwired: 2 in, 3 out]
        }
        n144 = for {
          tunnel: w12 -> [w22] mode=indexing
          shift-right: [w20] -> w9
          shift-left: w11 -> [w21]
          n145 = invoke class="SceneObject" method="Object.Remove Object"(reference=w21, "Child"=w22) -> (reference out=w20:refnum<vi>)  [unwired: 2 in, 3 out]
        }
        n146 = for {
          tunnel: w10 -> [w19] mode=indexing
          shift-right: [w17] -> w8
          shift-left: w9 -> [w18]
          n147 = invoke class="SceneObject" method="Object.Remove Object"(reference=w18, "Child"=w19) -> (reference out=w17:refnum<vi>)  [unwired: 2 in, 3 out]
        }
        n148 = Close Reference(reference=w8) -> ()  [unwired: 1 in, 1 out]
      }
      frame True {
      }
    }
  }
